vi "Check Setpoint.vi"(0 "Positions":dbl[](array[numeric]), 2 "Actions":T1, 7 "Limits":dbl[][](array[numeric]), 11 "Setpoints":dbl[](array[numeric]), 13 "Use Limits":bool) -> (8 "Setpoints Out":dbl[](array[numeric]))   [LabVIEW 2016]
uses:
  Stages Controls/Stage Actions.ctl
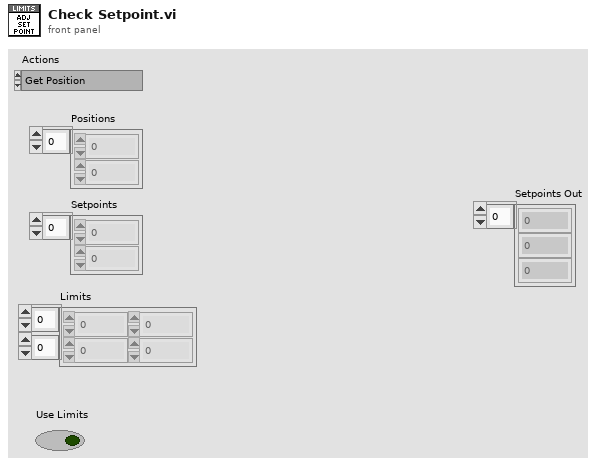
[diagram p1: front panel]
types:
  T1 = typedef "Stage Actions.ctl" = enum16{"Get Position", "MVR", "MOVE", "HALT", "ONTARGET", "ERROR", "REFERENCE", "INIT", "VELOCITY", "STATUS", "EXIT", "HOME", "ZEROPOS", "NANOPOS", "ANALOG", "QUIT"}
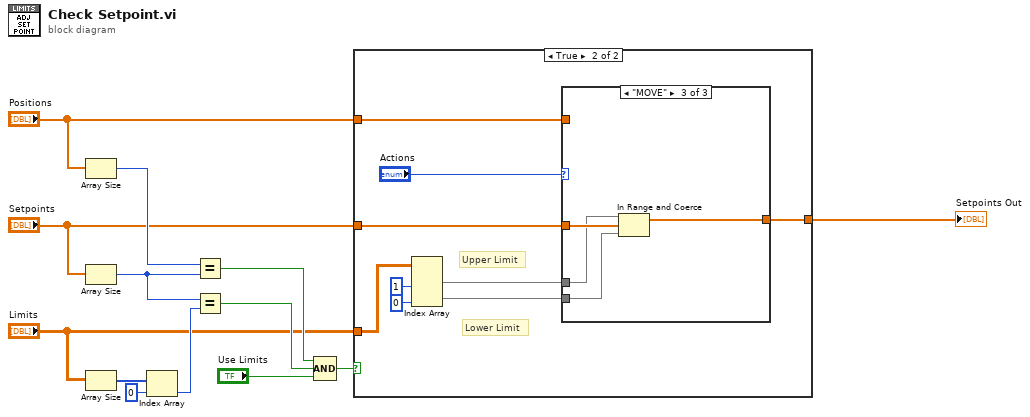
[diagram p0: block diagram]
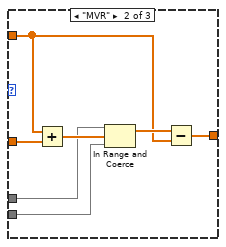
[diagram p4: hidden frame]
diagram:
  n1 = Array Size(array="Positions") -> (size(s)=w11:i32)
  n2 = Array Size(array="Setpoints") -> (size(s)=w9:i32)
  n3 = Array Size(array="Limits") -> (size(s)=w13:i32[])
  n4 = Index Array(array=w13, index=0) -> (element=w10:i32)
  n5 = Equal?(x=w11, y=w9) -> (x = y?=w6:bool)
  n6 = Equal?(x=w9, y=w10) -> (x = y?=w7:bool)
  n7 = Compound Arithmetic op=AND(w6, w7, "Use Limits") -> (w8:bool)
  n8 = case shown="True" w8 {
    tunnel: "Limits" -> [_ w20]
    tunnel: "Setpoints" -> [w14 w22]
    tunnel: "Positions" -> [_ w21]
    tunnel: [w14 w15] -> w1
    frame False {
    }
    frame True {
      # "Upper Limit"
      # "Lower Limit"
      n9 = Index Array(array=w20, index (col) #1=1 ("disabled index (col)"), index (col) #2=0 ("index (col)")) -> (element #1=w17:dbl[], element #2=w16:dbl[])  [unwired: 2 in]
      n10 = case shown="\"MOVE\"" "Actions" {
        tunnel: w22 -> [w24 w31 w35]
        tunnel: w21 -> [_ w26 _]
        tunnel: w17 -> [_ w29 w34]
        tunnel: w16 -> [_ w28 w33]
        tunnel: [w24 w25 w32] -> w15
        frame Default {
        }
        frame "MVR" {
          n11 = Add(x=w26, y=w31) -> (x+y=w30:dbl[])
          n12 = In Range and Coerce(upper limit=w29, x=w30, lower limit=w28) -> (coerced(x)=w27:dbl[])  [unwired: 1 out]
          n13 = Subtract(x=w27, y=w26) -> (x-y=w25:dbl[])
        }
        frame "MOVE" {
          n14 = In Range and Coerce(upper limit=w34, x=w35, lower limit=w33) -> (coerced(x)=w32:dbl[])  [unwired: 1 out]
        }
      }
    }
  }
  "Setpoints Out" <- w1
